vi "Save_MES_Log.vi"(0 "XML File Path":path caption="XML文件路径", 1 "SerialNumber":string, 2 "StatusCode":string, 3 "XML Input":string caption="XML输入", 4 "CELL":string) -> (6 "XML File Path(duplicate)":path caption="XML文件路径（副本）", 7 "XML String":string caption="XML字符串")   [LabVIEW 2018]
panel:
  in  "XML Encoding":string caption="XML编码"
  in  "Standalone? (T)":bool=TRUE caption="独立？(T)"
  in  "Prompt":string="选择XML文件路径" caption="提示"
  out "error out":errorcluster caption="错误输出"
  in  "error in (no error)":errorcluster caption="错误输入（无错误）"
  # "\\\\cngugmes01\\Shopfloor\\Temp\\HuaweiData\\L18HipotData"
  # "pass"
  # "<?xml version=\"1.0\" encoding=\"utf-8\" standalone=\"no\" ?>\n<vCheckTester xmlns:xsi=\"http://www.w3.org/2001/XMLSchema-instance\" xmlns:xsd=\"http://www.w3.org/2001/XMLSchema\" Version=\"4.0\" WorkOrderNumber=\"\" xmlns=\"Valor.vCheckTester.xsd\" OperatorNumber=\"\">\n<Unit Timestamp=\"2021-04-17T10:09:51\" SerialNumber=\"KF1118M4A00643\" DateTimeStart=\"2021-04-17T10:09:39\" DateTimeEnd=\"2021-04-17T10:09:51\" xmlns=\"Valor.vCheckTester.xsd\" StatusCode=\"PASS\">\n<Measurement DateTime=\"2021-04-17T10:09:51\" MeasurementUnit=\"AC(mA)\" LowerLimit=\"0.3\" UpperLimit=\"5\" ValueUnit=\"Double\" xmlns=\"Valor.vCheckTester.xsd\" Value=\"1.207999\" Name=\"AC\" StatusCode=\"PASS\" />\n<Measurement DateTime=\"2021-04-17T10:09:51\" MeasurementUnit=\"IR(Mohm)\" LowerLimit=\"100\" UpperLimit=\"0\" ValueUnit=\"Double\" xmlns=\"Valor.vCheckTester.xsd\" Value=\"50000000.000000\" Name=\"IR\" StatusCode=\"PASS\" />\n<Header TestProgramName=\"HW\" TestHeadNumber=\"HW\" TestProgramVersion=\"V1.0.0\" TestHeadType=\"Testser Information\" TestFixtureNumber=\"00001\"/>\n</Unit>\n</vCheckTester>"
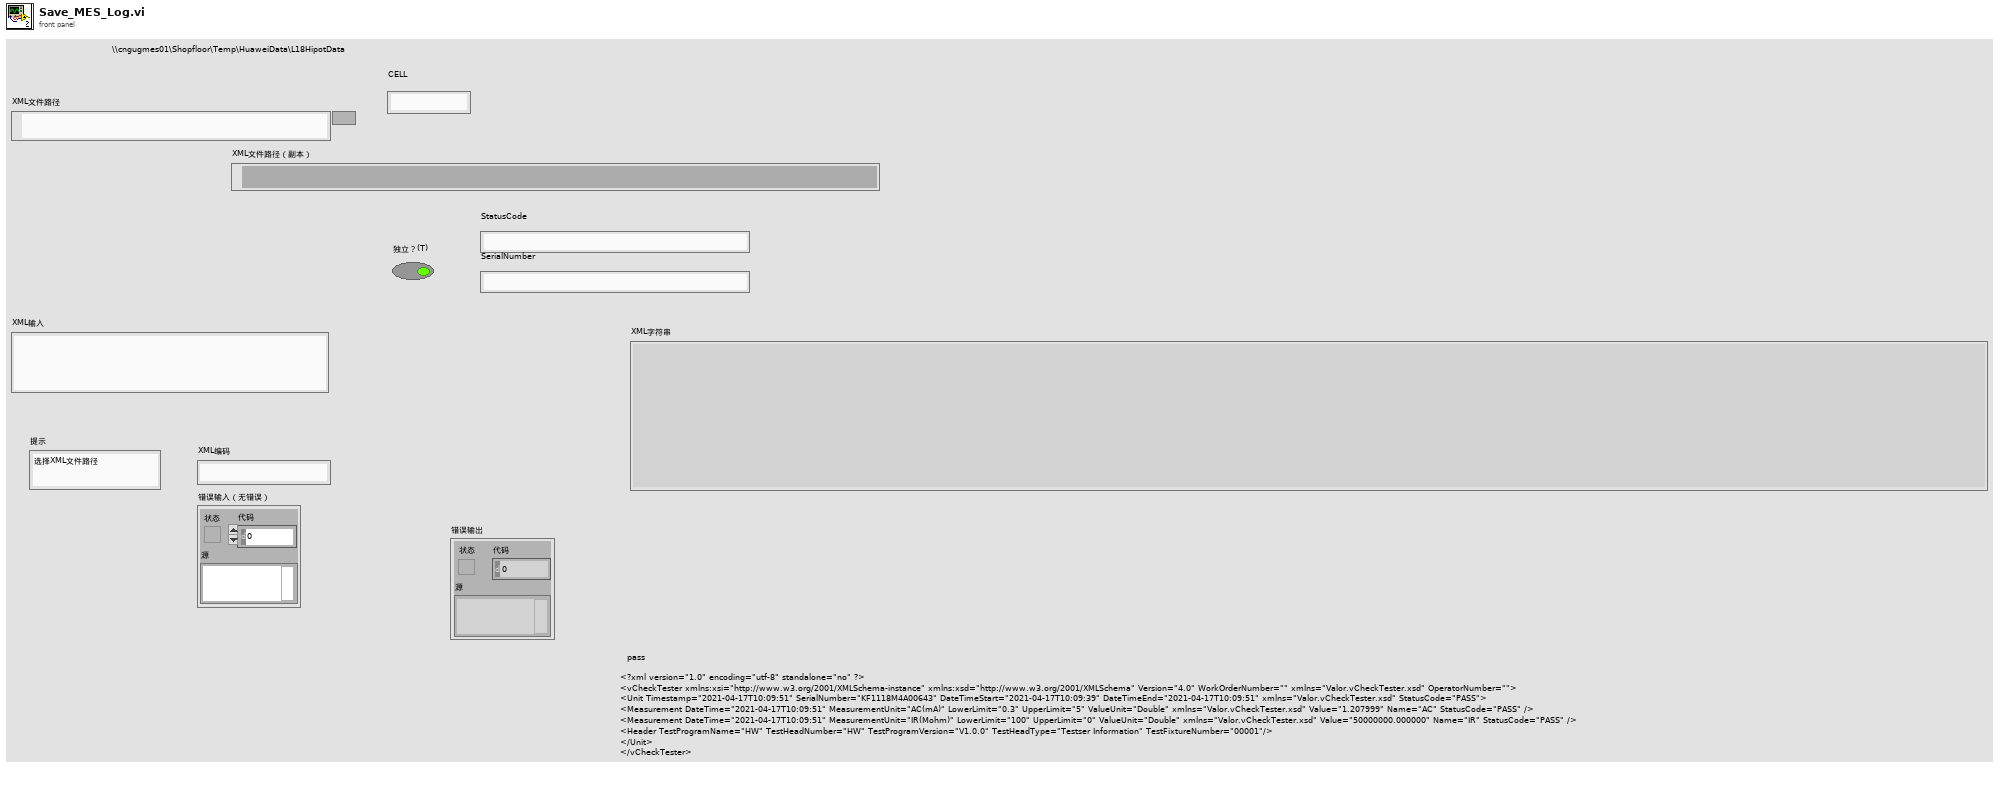
[diagram p1: front panel]
types:
  T1 = enum16{"open", "open or create", "create or replace", "create", "open (read only)"}
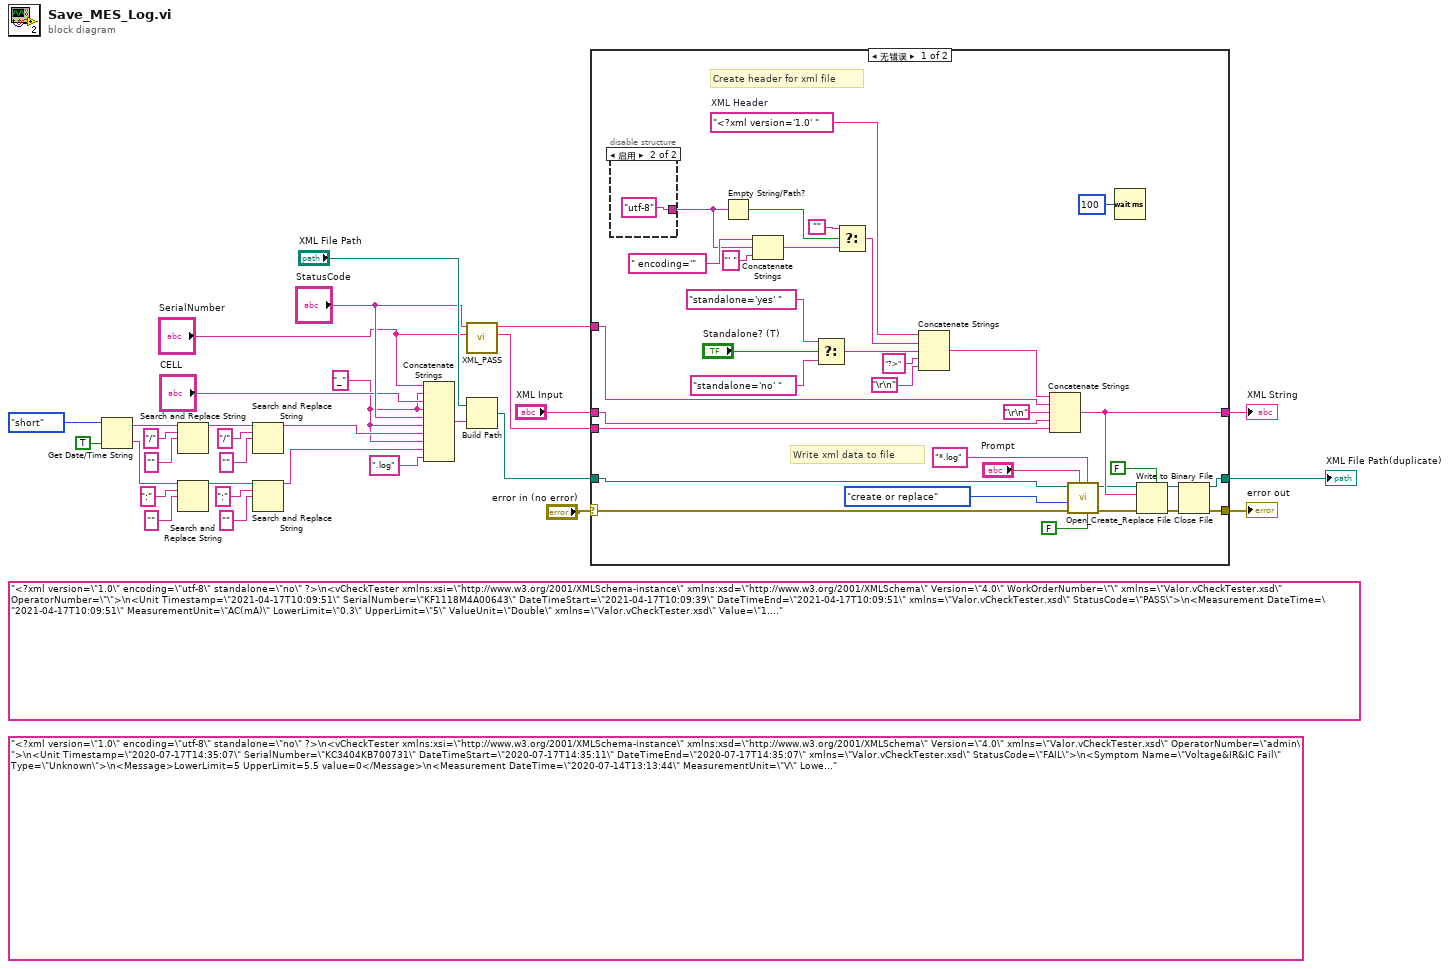
[diagram p0: block diagram]
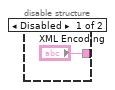
[diagram p2: hidden frame]
diagram:
  w2 = "_"
  (unwired) "<?xml version=\"1.0\" encoding=\"utf-8\" standalone=\"no\" ?>\n<vCheckTester xmlns:xsi=\"http://www.w3.org/2001/XMLSchema-instance\" xmlns:xsd=\"http://www.w3.org/2001/XMLSchema\" Version=\"4.0\" xmlns=\"Valor.vCheckTester.xsd\" OperatorNumber=\"admin\">\n<Unit Timestamp=\"2020-07-17T14:35:07\" SerialNumber=\"KC3404KB700731\" DateTimeStart=\"2020-07-17T14:35:11\" DateTimeEnd=\"2020-07-17T14:35:07\" xmlns=\"Valor.vCheckTester.xsd\" StatusCode=\"FAIL\">\n<Symptom Name=\"Voltage&IR&IC Fail\" Type=\"Unknown\">\n<Message>LowerLimit=5 UpperLimit=5.5 value=0</Message>\n<Measurement DateTime=\"2020-07-14T13:13:44\" MeasurementUnit=\"V\" LowerLimit=\"5\" UpperLimit=\"5.5\" ValueUnit=\"Double\" xmlns=\"Valor.vCheckTester.xsd\" Value=\"5.332\" Name=\"Read Voltage\" StatusCode=\"PASS\" />\n<Measurement DateTime=\"2020-07-17T14:35:07\" MeasurementUnit=\"V\" LowerLimit=\"5\" UpperLimit=\"5.5\" ValueUnit=\"Double\" xmlns=\"Valor.vCheckTester.xsd\" Value=\"5.199\" Name=\"Read Voltage\" StatusCode=\"FAIL\" />\n<Measurement DateTime=\"2020-07-14T13:13:44\" MeasurementUnit=\"V\" LowerLimit=\"5\" UpperLimit=\"5.5\" ValueUnit=\"Double\" xmlns=\"Valor.vCheckTester.xsd\" Value=\"5.332\" Name=\"Read Voltage\" StatusCode=\"PASS\" />\n</Symptom>\n<Header TestFixtureNumber=\"FIX-0003670618\"/>\n</Unit>\n</vCheckTester>\n"
  (unwired) "<?xml version=\"1.0\" encoding=\"utf-8\" standalone=\"no\" ?>\n<vCheckTester xmlns:xsi=\"http://www.w3.org/2001/XMLSchema-instance\" xmlns:xsd=\"http://www.w3.org/2001/XMLSchema\" Version=\"4.0\" WorkOrderNumber=\"\" xmlns=\"Valor.vCheckTester.xsd\" OperatorNumber=\"\">\n<Unit Timestamp=\"2021-04-17T10:09:51\" SerialNumber=\"KF1118M4A00643\" DateTimeStart=\"2021-04-17T10:09:39\" DateTimeEnd=\"2021-04-17T10:09:51\" xmlns=\"Valor.vCheckTester.xsd\" StatusCode=\"PASS\">\n<Measurement DateTime=\"2021-04-17T10:09:51\" MeasurementUnit=\"AC(mA)\" LowerLimit=\"0.3\" UpperLimit=\"5\" ValueUnit=\"Double\" xmlns=\"Valor.vCheckTester.xsd\" Value=\"1.207999\" Name=\"AC\" StatusCode=\"PASS\" />\n<Measurement DateTime=\"2021-04-17T10:09:51\" MeasurementUnit=\"IR(Mohm)\" LowerLimit=\"100\" UpperLimit=\"0\" ValueUnit=\"Double\" xmlns=\"Valor.vCheckTester.xsd\" Value=\"50000000.000000\" Name=\"IR\" StatusCode=\"PASS\" />\n<Header TestProgramName=\"HW\" TestHeadNumber=\"HW\" TestProgramVersion=\"V1.0.0\" TestHeadType=\"Testser Information\" TestFixtureNumber=\"00001\"/>\n</Unit>\n</vCheckTester>"
  n1 = Get Date/Time String(date format (0)=enum16{"short", "long", "abbreviated"}."short" ("日期格式(0)"), want seconds? (F)=TRUE ("需要秒？(F)")) -> (date string=w18:string, time string=w21:string)  [unwired: 1 in]
  n2 = Search and Replace String(input string=w18, search string="/" ("搜索字符串"), replace string="" ("替换字符串(\"\")")) -> (result string=w19:string)  [unwired: 5 in, 3 out]
  n3 = Search and Replace String(input string=w21, search string=":" ("搜索字符串"), replace string="" ("替换字符串(\"\")")) -> (result string=w20:string)  [unwired: 5 in, 3 out]
  n4 = Search and Replace String(input string=w19, search string="/" ("搜索字符串"), replace string="" ("替换字符串(\"\")")) -> (result string=w7:string)  [unwired: 5 in, 3 out]
  n5 = Search and Replace String(input string=w20, search string=":" ("搜索字符串"), replace string="" ("替换字符串(\"\")")) -> (result string=w6:string)  [unwired: 5 in, 3 out]
  n6 = Concatenate Strings("SerialNumber", w2, "CELL", w2, "StatusCode", w2, w7, w2, w6, ".log" ("字符串")) -> (w23:string)
  n7 = call "XML_PASS.vi"("SerialNumber"="SerialNumber", "StatusCode"="StatusCode") -> ("字符串"=w25:string, "字符串 2"=w26:string)  [unwired: 8 in]
  n8 = Build Path(base path="XML File Path", name or relative path=w23) -> (appended path=w5:path)
  n9 = case shown="无错误" "error in (no error)" {
    selector: "error in (no error)" -> [w47 w70]
    tunnel: [w48 w70] -> w30
    tunnel: "XML Input" -> [w50 w69]
    tunnel: [w46 w69] -> w28
    tunnel: [w45 w68] -> w27
    tunnel: w5 -> [w49 w68]
    tunnel: w26 -> [w43 _]
    tunnel: w25 -> [w42 _]
    frame No Error {
      w65 = "<?xml version='1.0' "  # XML Header
      # "Write xml data to file"
      # "Create header for xml file"
      n10 = disable-structure shown="启用" {
        disable-tunnel: ["XML Encoding" "utf-8" ("XML Encoding")] -> w58
        frame Disabled {
        }
        frame Enabled {
        }
      }
      n11 = Empty String/Path?(string/path=w58) -> (empty?=w57:bool)
      n12 = Concatenate Strings(" encoding='", w58, "' " ("Substring")) -> (w56:string)
      n13 = Select(t="standalone='yes' " ("Substring"), s="Standalone? (T)", f="standalone='no' " ("Substring")) -> (s? t:f=w51:string)
      n14 = Select(t="", s=w57, f=w56) -> (s? t:f=w54:string)
      n15 = Concatenate Strings(w65, w54, w51, "?>" ("Substring"), "\r\n") -> (w62:string)
      n16 = Concatenate Strings(w62, w43, "\r\n", w50, w42) -> (w46:string)
      n17 = call <vilib>:"Open_Create_Replace File.vi"("advisory dialog? (display:T)"=FALSE, "pattern"="*.log", "prompt"="Prompt", "error in (no error)"=w47, "function (open:0)"=T1."create or replace", "file path"=w49) -> ("error out"=w40:errorcluster, "refnum"=w38:refnum<file>)  [unwired: 2 in, 2 out]
      n18 = Wait (ms)(milliseconds to wait=u32 100 ("等待时间（毫秒）")) -> ()  [unwired: 1 out]
      n19 = Write to Binary File(file (use dialog)=w38, data=w46, error in=w40, 5:FALSE ("prepend array or string size? (T)")) -> (refnum out=w36:refnum<file>, error out=w39:errorcluster)  [unwired: 3 out]
      n20 = Close File(refnum=w36, error in=w39) -> (path=w45:path, error out=w48:errorcluster)
    }
    frame Error {
    }
  }
  "error out" <- w30
  "XML String" <- w28
  "XML File Path(duplicate)" <- w27
